vi "Radar3.vi"() -> ()   [LabVIEW 2017]
panel:
  out "ping":bool
  in  "target coordinates":cluster{"X":i16, "Y":i16}={"X"=-23, "Y"=57}
  in  "stop":bool
  out "2D Picture":picture
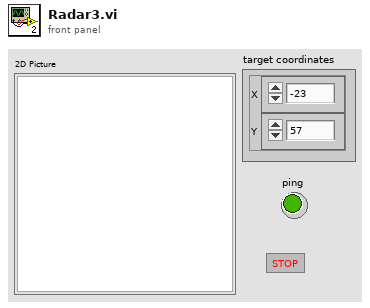
[diagram p1: front panel]
types:
  T1 = cluster{"maximum":dbl, "minimum":dbl, "clip to min":bool, "log?(F)":bool, "grid color":u32, "plot color":u32, "fmt and prec":cluster{"format":enum8{"Decimal", "Scientific", "Engineering", "Binary", "Octal", "Hex"}, "precision":u8}, "visible section":u16}
  T2 = cluster{"Width":u16, "Style":enum32{"Solid", "Dash", "Dot", "DashDot", "DashDotDot"}}
  T3 = typedef "imagedata.ctl" = cluster{"image type":i32, "image depth":i32, "image":u8[], "mask":u8[], "colors":u32[], "Rectangle":cluster{"left":i16, "top":i16, "right":i16, "bottom":i16}}
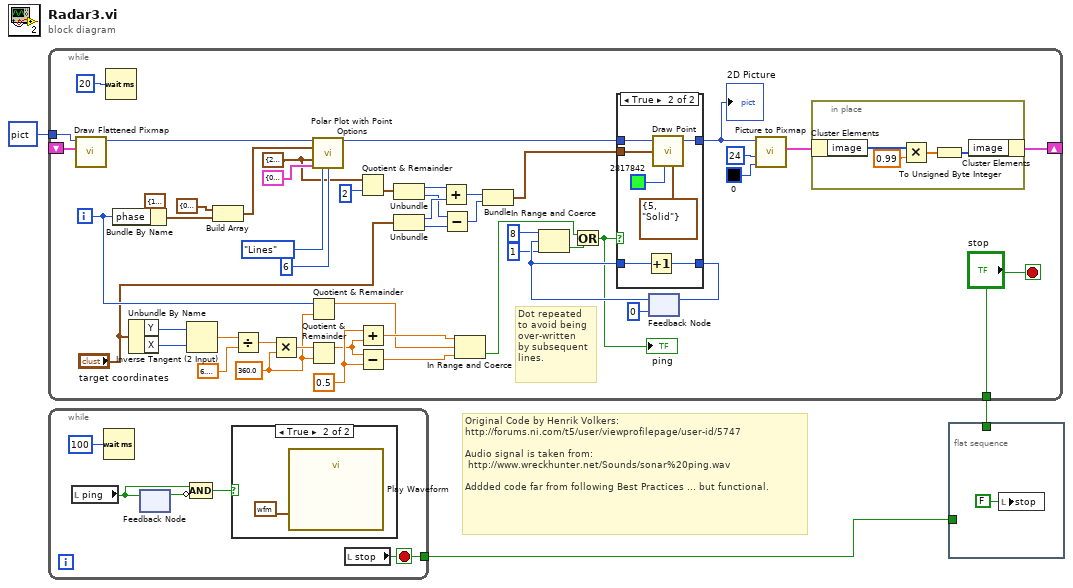
[diagram p0: block diagram]
diagram:
  # "Original Code by Henrik Volkers:\nhttp://forums.ni.com/t5/user/viewprofilepage/user-id/5747\n\nAudio signal is taken from:\n\thttp://www.wreckhunter.net/Sounds/sonar%20ping.wav\n\nAddded code far from following Best Practices ... but functional."
  n1 = while {
    shift-right: [w48] -> _
    shift-left: _ -> [w47]
    tunnel: picture data[5B] ("2D Picture") -> [w46]
    tunnel: ["stop"] -> w2
    i -> [w27]
    stop <- "stop" stop-if-true
    w34 = 0.5
    w26 = 360.0 ("y")
    w15 = cluster{"width":i16, "height":i16} {"width"=222, "height"=222} ("dimensions (w,h)")
    # "Dot repeated\nto avoid being\nover-written\nby subsequent\nlines."
    n2 = call <vilib>:"Draw Flattened Pixmap.vi"("image data"=w47, "picture"=w46) -> ("new picture"=w53:picture)  [unwired: 7 in]
    n3 = Wait (ms)(milliseconds to wait=u32 20) -> ()  [unwired: 1 out]
    n4 = Bundle By Name(cluster=cluster{"magnitude":dbl, "phase":dbl} {"magnitude"=100.0, "phase"=0.0}, "phase"=w27) -> (w44:cluster{"magnitude":dbl, "phase":dbl})
    n5 = Unbundle By Name("target coordinates") -> ("Y"=w37:i16, "X"=w36:i16)
    n6 = Inverse Tangent (2 Input)(1:w36, 2:w37) -> (0:w31:dbl)
    n7 = Build Array(cluster{"magnitude":dbl, "phase":dbl} {"magnitude"=0.0, "phase"=0.0}, w44) -> (w40:cluster{"magnitude":dbl, "phase":dbl}[])
    n8 = Divide(x=w31, y=6.283185307179586) -> (x/y=w30:dbl)
    n9 = Multiply(x=w30, y=w26) -> (x*y=w29:dbl)
    n10 = Quotient & Remainder(x=w27, y=w26) -> (x-y*floor(x/y)=w25:dbl)  [unwired: 1 out]
    n11 = Quotient & Remainder(x=w29, y=w26) -> (x-y*floor(x/y)=w28:dbl)  [unwired: 1 out]
    n12 = call <vilib>:"Polar Plot with Point Options.vi"("picture"=w53, "data array [mag, phase (deg)]"=w40, "dimensions (w,h)"=w15, "polar attributes"=T1 {"maximum"=0.0, "minimum"=0.0, "clip to min"=FALSE, "log?(F)"=FALSE, "grid color"=6710886, "plot color"=2465536, "fmt and prec"={"format"=enum."Decimal", "precision"=0}, "visible section"=8}, "Lines/Points"=enum16{"Lines", "Points"}."Lines", "Size"=u16 6) -> ("new picture"=w52:picture)  [unwired: 9 in]
    n13 = Quotient & Remainder(x=w15, y=i16 2) -> (floor(x/y)=w21:cluster{"width":i16, "height":i16})  [unwired: 1 out]
    n14 = Add(x=w34, y=w28) -> (x+y=w33:dbl)
    n15 = Subtract(x=w28, y=w34) -> (x-y=w32:dbl)
    n16 = Unbundle(w21) -> ("width"=w20:i16, "height"=w18:i16)
    n17 = Unbundle("target coordinates") -> ("X"=w19:i16, "Y"=w17:i16)
    n18 = Add(x=w20, y=w19) -> (x+y=w16:i16)
    n19 = Subtract(x=w18, y=w17) -> (x-y=w14:i16)
    n20 = In Range and Coerce(upper limit=w33, x=w25, lower limit=w32) -> (In Range?=w5:bool)  [unwired: 1 out]
    n21 = Bundle(w16, w14) -> (w13:cluster{i16, i16})  [unwired: 1 in]
    n22 = feedback #1(u8 0) -> (w9:u8)
    n23 = In Range and Coerce(upper limit=u8 8 ("y"), x=w9, lower limit=u8 1) -> (In Range?=w10:bool)  [unwired: 1 out]
    n24 = Or(x=w5, y=w10) -> (x .or. y?=w6:bool)
    "ping" <- w6
    n25 = case shown="True" w6 {
      tunnel: w52 -> [w54 w61]
      tunnel: [w54 w60] -> w38
      tunnel: w13 -> [_ w59]
      tunnel: [_ w56] -> w12
      tunnel: w9 -> [_ w55]
      frame False {
      }
      frame True {
        n26 = Increment(x=w55) -> (x+1=w56:u8)
        n27 = call <vilib>:"Draw Point.vi"("picture"=w61, "point(x,y)"=w59, "color(black)"=u32 2817842 ("plot color"), "pen"=T2 {"Width"=5, "Style"=enum."Solid"}) -> ("new picture"=w60:picture)  [unwired: 5 in]
      }
    }
    "2D Picture" <- w38
    n28 = feedback-in #1(w12) -> ()
    n29 = call <vilib>:"Picture to Pixmap.vi"("Background Color"=u32 0, "depth"=24, "picture"=w38) -> ("image data"=w49:T3)  [unwired: 7 in, 1 out]
    n30 = in-place {
      n31 = in-place-cluster #2(w49) -> ("image"=w65:u8[])
      n32 = Multiply(x=w65, y=0.99) -> (x*y=w63:dbl[])
      n33 = To Unsigned Byte Integer(number=w63) -> (unsigned 8bit integer=w62:u8[])
      n34 = in-place-cluster #2("image"=w62) -> (w48:T3)
    }
  }
  n35 = while {
    tunnel: [w67] -> w1
    stop <- w67 stop-if-true
    n36 = local read "ping"() -> (w70:bool)
    n37 = Wait (ms)(milliseconds to wait=u32 100) -> ()  [unwired: 1 out]
    n38 = feedback-in #3(w70) -> ()
    n39 = feedback #3() -> (w69:bool)  [unwired: 1 in]
    n40 = Compound Arithmetic op=AND(w70, invert w69) -> (w68:bool)
    n41 = case shown="True" w68 {
      frame False {
      }
      frame True {
        n42 = call "Play Waveform"("Data"=waveform(dbl) {"t0"=timestamp(0.15 s since 1904-01-01), "dt"=0.000125, "Y"=array[16000 elements]} ("output waveform")) -> ()  [unwired: 18 in, 1 out]
      }
    }
    n43 = local read "stop"() -> (w67:bool)
  }
  n44 = flat-sequence {
    tunnel: w2 -> [_]
    tunnel: w1 -> [_]
    frame #0 {
      n45 = local write "stop"(FALSE ("stop")) -> ()
    }
  }
